vi "read_temporal_calibration.vi"(8 "error in (no error)":errorcluster, 10 "Median Filtered Image":T1, 11 "Aquired Image":T1) -> (0 "error out":errorcluster, 1 "Other Bits Decoded":bool[](array[boolean]), 2 "Time Bits Decoded":bool[](array[boolean]))   [LabVIEW 2019]
uses:
  <vilib>/vision/Image Controls.llb/IMAQ Image.ctl
  ParametersGlobal.vi
  <vilib>/vision/NI_Vision_Development_Module.lvlib
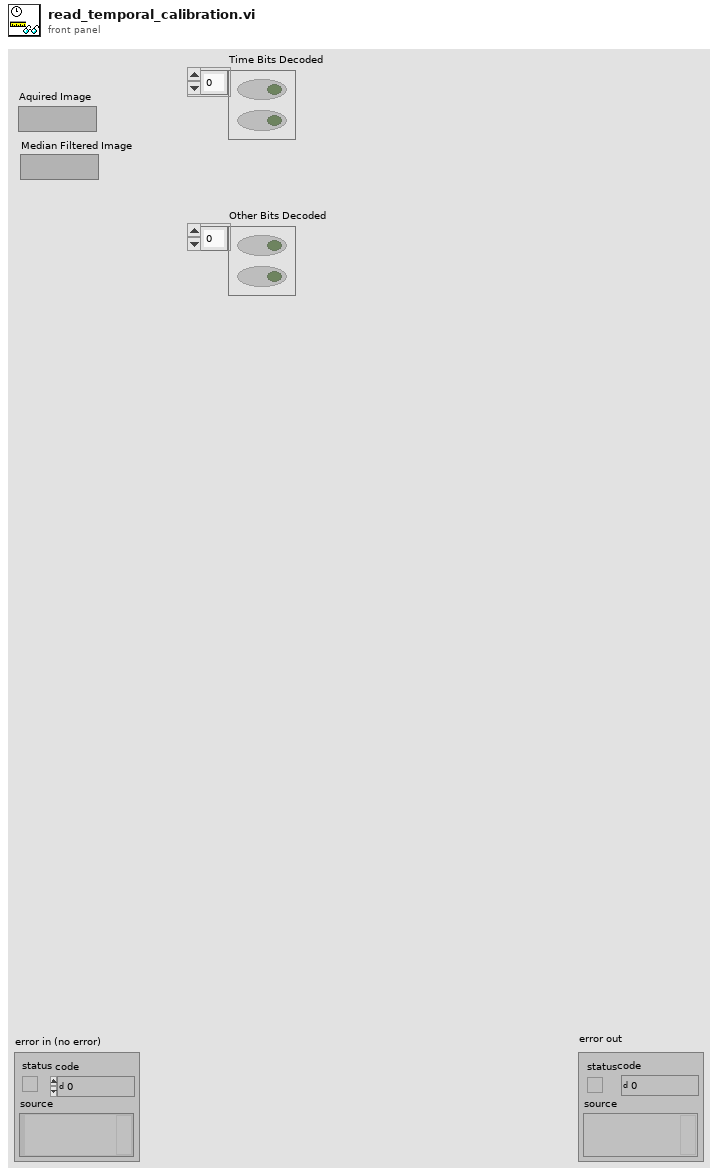
[diagram p1: front panel]
types:
  T1 = typedef "IMAQ Image.ctl" = refnum<image>
  T2 = typedef "Image Type" = u32
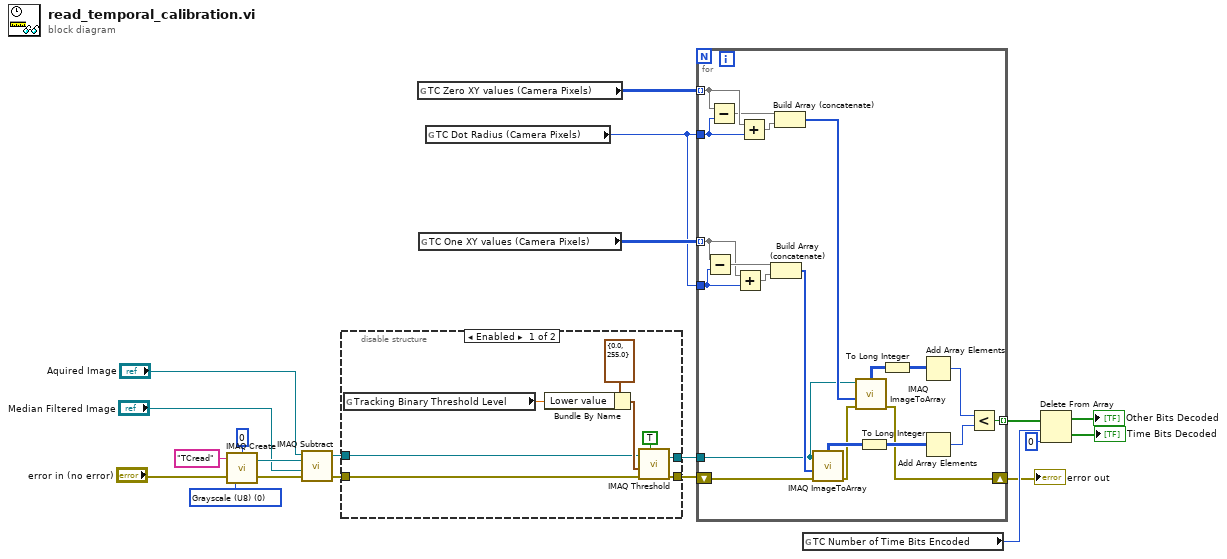
[diagram p0: block diagram]
diagram:
  w13 = T2 0 items=["Grayscale (U8)", "Grayscale (I16)", "Grayscale (SGL)", "Complex (CSG)", "RGB (U32)", "HSL (U32)", "RGB (U64)"] ("Image Type")
  n1 = call "IMAQ Create"("Border Size"=0, "Image Name"="TCread", "Image Type"=w13, "error in (no error)"="error in (no error)") -> ("New Image"=w8:T1, "error out"=w9:errorcluster)  [unwired: 1 in]
  n2 = call "IMAQ Subtract"("Image Src A"="Aquired Image", "Image Dst"=w8, "Image Src B"="Median Filtered Image", "error in (no error)"=w9) -> ("Image Dst Out"=w4:T1, "error out"=w5:errorcluster)  [unwired: 3 in]
  n3 = disable-structure shown="Enabled" {
    disable-tunnel: w5 -> [w26 w30]
    disable-tunnel: w4 -> [w25 w31]
    disable-tunnel: [w23 w30] -> w3
    disable-tunnel: [w22 w31] -> w2
    frame Enabled {
      n4 = global read "ParametersGlobal.vi" "Tracking Binary Threshold Level"() -> (w27:sgl)
      n5 = Bundle By Name(cluster=cluster{"Lower value":sgl, "Upper value":sgl} {"Lower value"=0.0, "Upper value"=255.0} ("Range"), "Lower value"=w27) -> (w29:cluster{"Lower value":sgl, "Upper value":sgl})
      n6 = call "IMAQ Threshold"("Keep/Replace Value (Replace)"=TRUE, "error in (no error)"=w26, "Range"=w29, "Image Src"=w25) -> ("error out"=w23:errorcluster, "Image Dst Out"=w22:T1)  [unwired: 6 in]
    }
    frame Disabled {
    }
  }
  n7 = global read "ParametersGlobal.vi" "TC Zero XY values (Camera Pixels)"() -> (w17:i32[][])
  n8 = global read "ParametersGlobal.vi" "TC One XY values (Camera Pixels)"() -> (w16:i32[][])
  n9 = global read "ParametersGlobal.vi" "TC Dot Radius (Camera Pixels)"() -> (w15:i32)
  n10 = for {
    tunnel: w15 -> [w43]
    tunnel: [w52] -> w1 mode=indexing
    shift-right: [w33] -> w14
    shift-left: w3 -> [w51]
    tunnel: w16 -> [w36] mode=indexing
    tunnel: w17 -> [w44] mode=indexing
    tunnel: w15 -> [w37]
    tunnel: w2 -> [w32]
    n11 = Subtract(x=w36, y=w37) -> (x-y=w39:i32[])
    n12 = Subtract(x=w44, y=w43) -> (x-y=w42:i32[])
    n13 = Add(x=w36, y=w37) -> (x+y=w38:i32[])
    n14 = Add(x=w44, y=w43) -> (x+y=w41:i32[])
    n15 = Build Array (concatenate)(w39, w38) -> (w35:i32[])
    n16 = Build Array (concatenate)(w42, w41) -> (w40:i32[])
    n17 = call "IMAQ ImageToArray"("error in (no error)"=w51, "Optional Rectangle"=w35, "Image"=w32) -> ("error out"=w34:errorcluster, "Image Pixels (U8)"=w48:u8[][])  [unwired: 1 in, 3 out]
    n18 = call "IMAQ ImageToArray"("error in (no error)"=w34, "Optional Rectangle"=w40, "Image"=w32) -> ("error out"=w33:errorcluster, "Image Pixels (U8)"=w50:u8[][])  [unwired: 1 in, 3 out]
    n19 = To Long Integer(number=w48) -> (32bit integer=w47:i32[][])
    n20 = To Long Integer(number=w50) -> (32bit integer=w49:i32[][])
    n21 = Add Array Elements(numeric array=w49) -> (sum=w46:i32)
    n22 = Add Array Elements(numeric array=w47) -> (sum=w45:i32)
    n23 = Less?(x=w46, y=w45) -> (x < y?=w52:bool)
  }
  "error out" <- w14
  n24 = global read "ParametersGlobal.vi" "TC Number of Time Bits Encoded"() -> (w18:i32)
  n25 = Delete From Array(array=w1, length=w18, index=0) -> (deleted portion=→"Time Bits Decoded":bool[], array with subset deleted=→"Other Bits Decoded":bool[])
